vi "PWM to CAN.vi"(8 "cluster manipulator 2":T3, 9 "serwa i pompa":T1={"lewy tyl "=TRUE, "prawy tyl "=TRUE, "lewy przod "=TRUE, "œrodek"=TRUE, "prawy przod "=TRUE, "serwo 3"=TRUE, "serwo 4 "=TRUE, "przekaznik"=TRUE}, 11 "MANIPULATOR ID 3":u32) -> (1 "array of cans":T2[](array[typedef]) {"type" items=["CAN Data", "CAN Remote"]; "identifier" format="%.0x"}, 2 "druga ramka manipulator":T2 {"type" items=["CAN Data", "CAN Remote"]; "identifier" format="%.0x"}, 3 "Pierwsza ramka manipulator":T2 {"type" items=["CAN Data", "CAN Remote"]; "identifier" format="%.0x"})   [LabVIEW 2014]
uses:
  CANFrameControl.ctl
  klapki.ctl
panel:
  out "unsigned 8bit integer":u8
  out "0, 1":i16[](array[numeric])
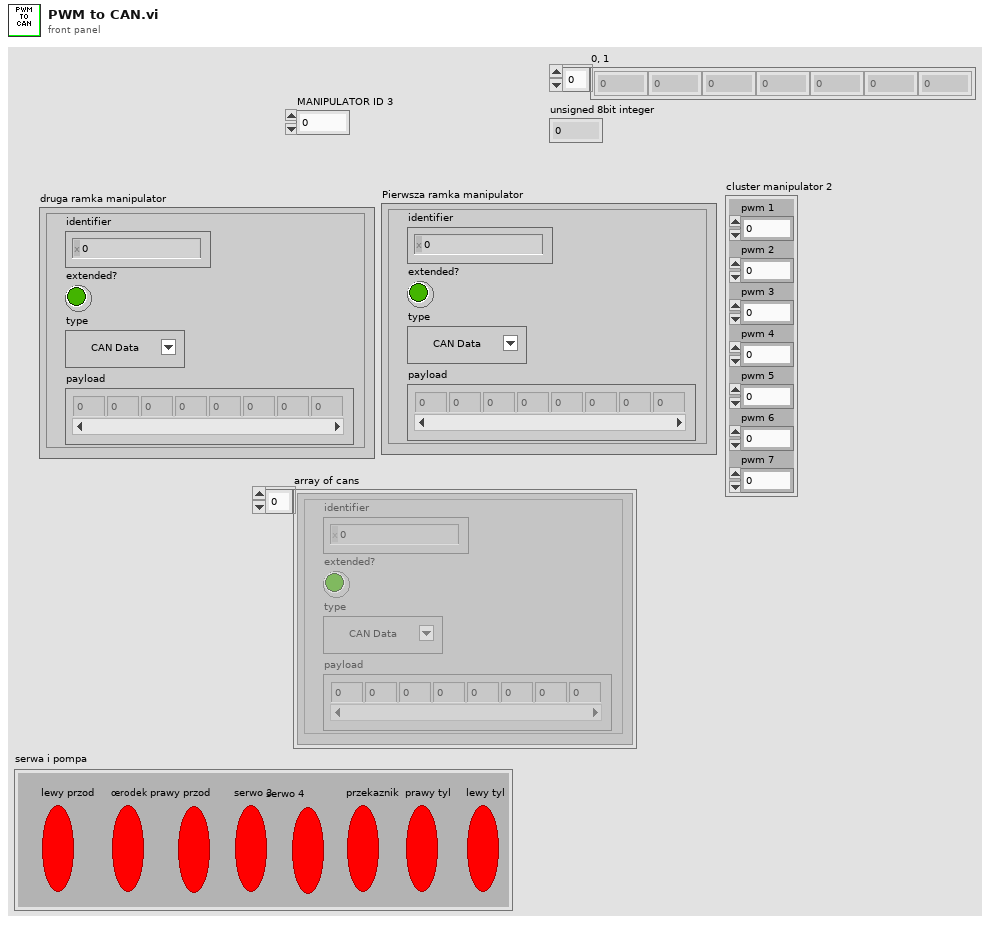
[diagram p1: front panel]
types:
  T1 = typedef "klapki.ctl" = cluster{"lewy tyl ":bool, "prawy tyl ":bool, "lewy przod ":bool, "œrodek":bool, "prawy przod ":bool, "serwo 3":bool, "serwo 4 ":bool, "przekaznik":bool}
  T2 = typedef "CANFrameControl.ctl" = cluster{"identifier":u32, "extended?":bool, "type":u8, "payload":u8[]}
  T3 = cluster{"pwm 1":dbl, "pwm 2":dbl, "pwm 3":dbl, "pwm 4":dbl, "pwm 5":dbl, "pwm 6":dbl, "pwm 7":dbl}
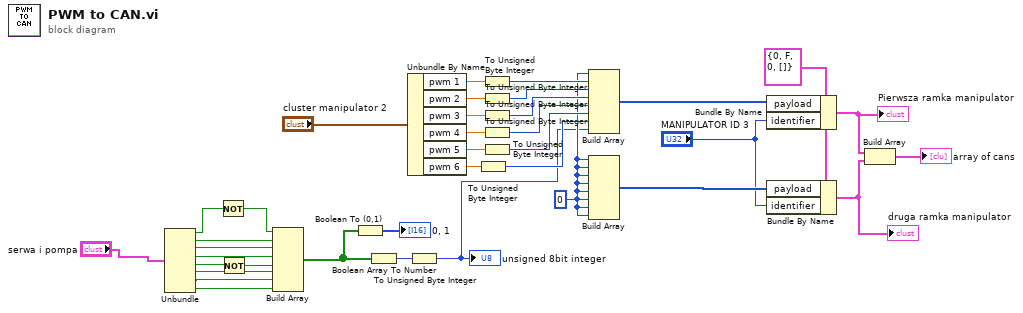
[diagram p0: block diagram]
diagram:
  w16 = u8 0
  w30 = T2 {"identifier"=0, "extended?"=FALSE, "type"=0, "payload"=[]} ("CAN frame 2")
  n1 = Unbundle("serwa i pompa") -> ("lewy tyl"=w2:bool, "prawy tyl"=w6:bool, "lewy przod"=w15:bool, "œrodek"=w14:bool, "prawy przod"=w4:bool, "serwo 3"=w10:bool, "serwo 4"=w5:bool, "przekaznik"=w9:bool)
  n2 = Not(x=w2) -> (.not. x?=w1:bool)
  n3 = Not(x=w4) -> (.not. x?=w3:bool)
  n4 = Build Array(w1, w6, w15, w14, w3, w10, w5, w9) -> (w7:bool[])
  n5 = Boolean To (0,1)(Boolean=w7) -> (0, 1=→"0, 1":i16[])
  n6 = Boolean Array To Number(Boolean array=w7) -> (number=w13:u32)
  n7 = Unbundle By Name("cluster manipulator 2") -> ("pwm 1"=w35:dbl, "pwm 2"=w34:dbl, "pwm 3"=w33:dbl, "pwm 4"=w32:dbl, "pwm 5"=w31:dbl, "pwm 6"=w24:dbl)
  n8 = To Unsigned Byte Integer(number=w13) -> (unsigned 8bit integer=w11:u8)
  "unsigned 8bit integer" <- w11
  n9 = To Unsigned Byte Integer(number=w24) -> (unsigned 8bit integer=w18:u8)
  n10 = To Unsigned Byte Integer(number=w35) -> (unsigned 8bit integer=w23:u8)
  n11 = To Unsigned Byte Integer(number=w34) -> (unsigned 8bit integer=w22:u8)
  n12 = To Unsigned Byte Integer(number=w33) -> (unsigned 8bit integer=w21:u8)
  n13 = To Unsigned Byte Integer(number=w32) -> (unsigned 8bit integer=w20:u8)
  n14 = To Unsigned Byte Integer(number=w31) -> (unsigned 8bit integer=w19:u8)
  n15 = Build Array(w16, w23, w22, w21, w20, w19, w18, w11) -> (w17:u8[])
  n16 = Build Array(w16, w16, w16, w16, w16, w16, w16, w16) -> (w29:u8[])
  n17 = Bundle By Name(cluster=w30, "payload"=w17, "identifier"="MANIPULATOR ID 3") -> (w27:T2)
  "Pierwsza ramka manipulator" <- w27
  n18 = Bundle By Name(cluster=w30, "payload"=w29, "identifier"="MANIPULATOR ID 3") -> (w26:T2)
  "druga ramka manipulator" <- w26
  n19 = Build Array(w27, w26) -> (→"array of cans":T2[])
